vi "MMEM_LOAD.vi"(0 "VISA IN":refnum<visa-resource-name>, 2 "FileName":string, 5 "error in":errorcluster, 7 "FileType":string="CSA") -> (14 "VISA Out":refnum<visa-resource-name>, 19 "error out":errorcluster)   [LabVIEW 2018, in "PNA-X.lvlib"]
doc: "MMEMory:LOAD[:<char>] <file> \n1610\n\n(Write-only) Loads the specified file. Learn about File Types \nParameters \n<char> The type of file to load. Choose from: \nSTATe - Instrument states (.sta) \nCORRection - Calibration Data (.cal) \nCSARchive - Instrument state and calibration data (.csa) \nCSTate - Instrument state and link to Calibration data (.cst) \nIf <char> is unspecified, the extension must be included in the filename. \nIf an extension is specified in <file> that does not agree with <char> then no \naction is taken. \n<file> String - Name of the file to be loaded. See Specifying Path Names \nExamples MMEM:LOAD 'MyFile.cst' \nmmemory:load:state 'MyInstState' \nQuery Syntax Not applicable \nDefault Not applicable"
uses:
  PNA-X.lvlib
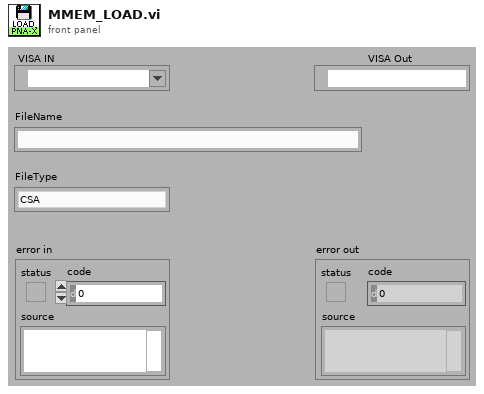
[diagram p1: front panel]
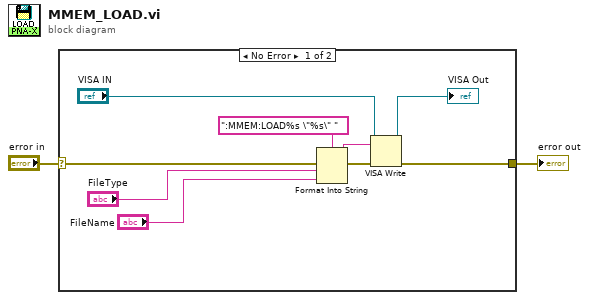
[diagram p0: block diagram]
diagram:
  n1 = case shown="No Error" "error in" {
    selector: "error in" -> [w11 w12]
    tunnel: [w6 w12] -> w1
    frame No Error {
      n2 = Format Into String(format string=":MMEM:LOAD%s \"%s\" " ("Cmdline"), error in=w11, "FileType", "FileName") -> (resulting string=w9:string, error out=w10:errorcluster)  [unwired: 1 in]
      n3 = VISA Write(VISA resource name="VISA IN", write buffer=w9, error in (no error)=w10) -> (VISA resource name out=→"VISA Out":refnum<visa-resource-name>, error out=w6:errorcluster)  [unwired: 1 out]
    }
    frame Error {
    }
  }
  "error out" <- w1
